vi "Enter Firing Head Info.vi"(7 "error in (no error)":errorcluster) -> (0 "error out":errorcluster, 1 "Abort Test?":bool, 2 "Serial # Out":string, 3 "Model # Out":string)   [LabVIEW 2018]
uses:
  Instrumentation/Door Status Global Variable.vi
panel:
  in  "Model #":string
  in  "Abort Test":bool
  in  "Serial #":string
  in  "Continue":bool
  # "Enter the following information\nfor the firing head:"
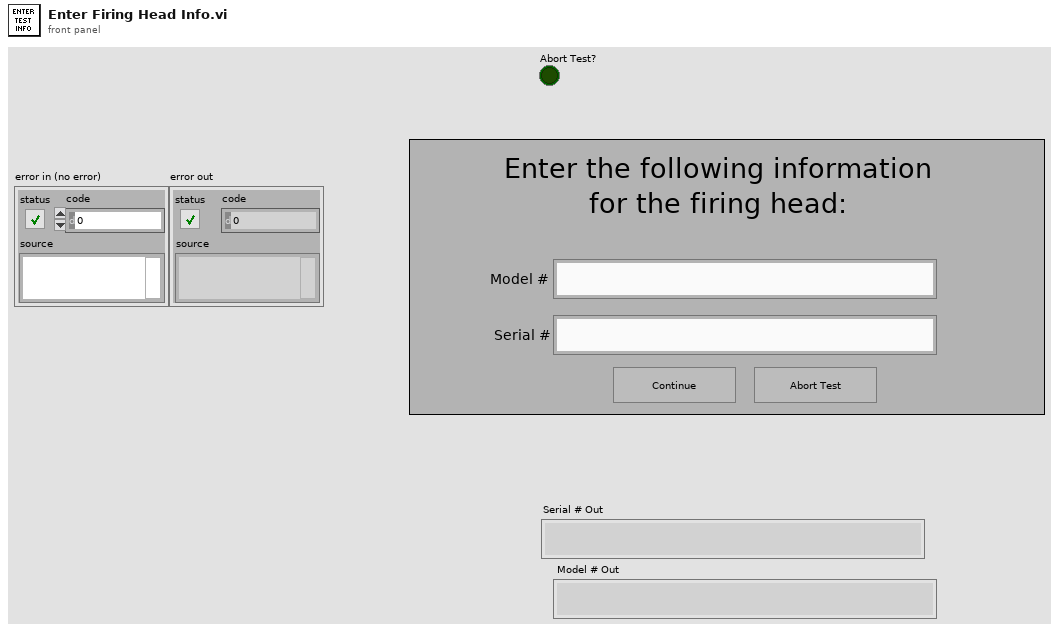
[diagram p1: front panel]
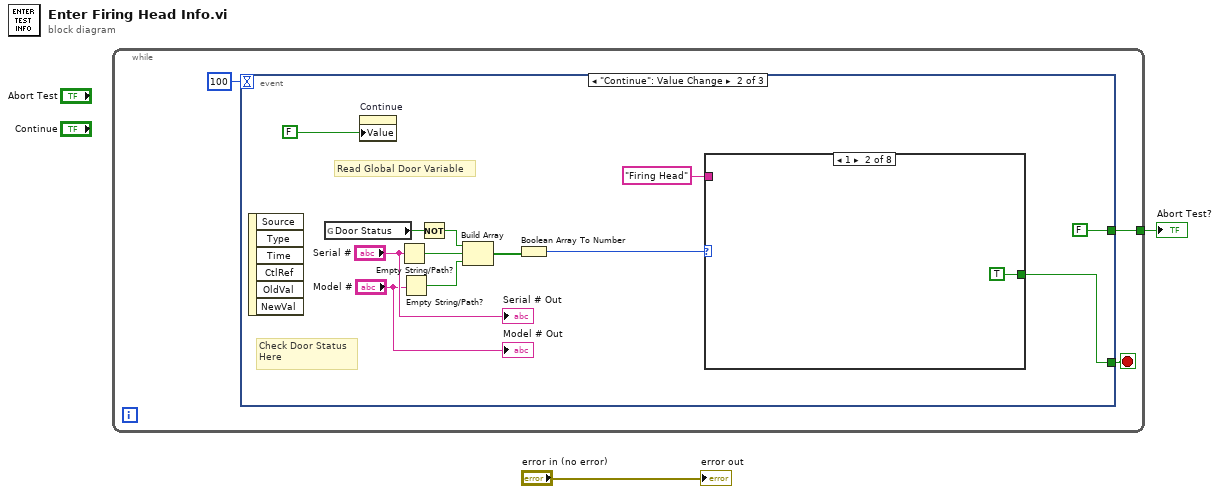
[diagram p0: block diagram]
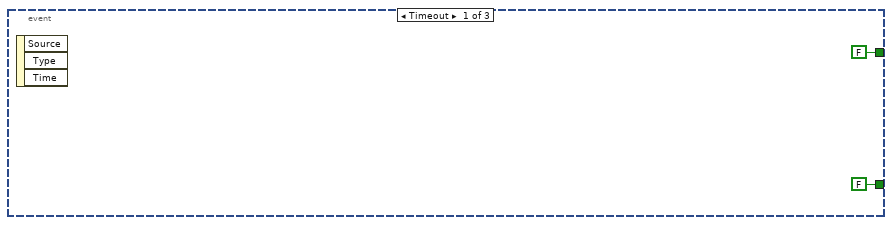
[diagram p2: hidden frame]
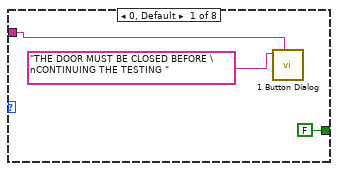
[diagram p3: hidden frame]
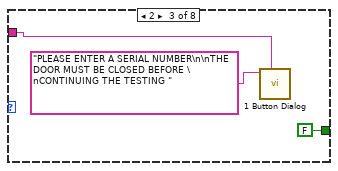
[diagram p4: hidden frame]
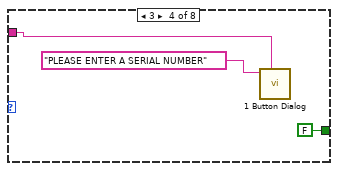
[diagram p5: hidden frame]
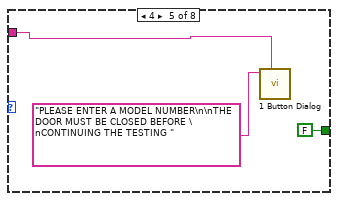
[diagram p6: hidden frame]
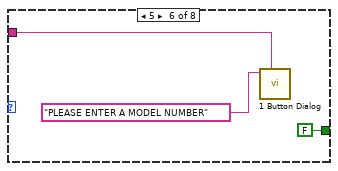
[diagram p7: hidden frame]
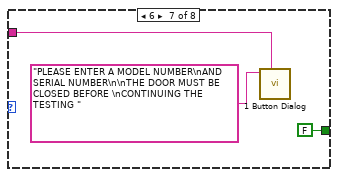
[diagram p8: hidden frame]
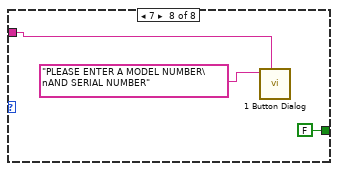
[diagram p9: hidden frame]
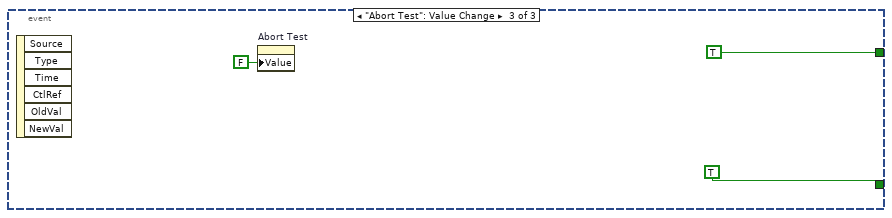
[diagram p10: hidden frame]
diagram:
  n1 = while {
    tunnel: [w4] -> w1
    stop <- w5 stop-if-true
    n2 = event shown="[1] \"Continue\": Value Change" {
      selector: _ -> [_ _ _]
      dyn-events: _ -> [_ _ _]
      timeout: 100 -> [_ _ _]
      tunnel: [FALSE ("Global Stop?") w12 TRUE] -> w5
      tunnel: [FALSE FALSE TRUE] -> w4
      event Timeout {
        n3 = event-data() -> ()  [unwired: 1 in, 3 out]
      }
      event "Continue": Value Change {
        # "Read Global Door Variable"
        # "Check Door Status\nHere"
        n4 = event-data() -> ()  [unwired: 1 in, 6 out]
        n5 = global read "Door Status Global Variable.vi" "Door Status"() -> (w9:bool)
        n6 = property on="Continue" class="Bool (strict)"("Value"=FALSE ("OK")) -> ()  [unwired: 2 in, 2 out]
        n7 = Empty String/Path?(string/path="Serial #") -> (empty?=w14:bool)
        n8 = Empty String/Path?(string/path="Model #") -> (empty?=w13:bool)
        n9 = Not(x=w9) -> (.not. x?=w8:bool)
        n10 = Build Array(w8, w14, w13) -> (w18:bool[])
        n11 = Boolean Array To Number(Boolean array=w18) -> (number=w17:u32)
        n12 = case shown="1" w17 {
          tunnel: [FALSE ("Global Stop?") TRUE ("Global Stop?") FALSE ("Global Stop?") FALSE ("Global Stop?") FALSE ("Global Stop?") FALSE ("Global Stop?") FALSE ("Global Stop?") FALSE ("Global Stop?")] -> w12
          tunnel: "Firing Head" ("Title") -> [w21 _ w25 w28 w31 w34 w37 w40]
          frame 0, Default {
            n13 = call "1 Button Dialog.vi"("Title"=w21, "Dialog Message"="THE DOOR MUST BE CLOSED BEFORE \nCONTINUING THE TESTING ") -> ()  [unwired: 8 in, 2 out]
          }
          frame 1 {
          }
          frame 2 {
            n14 = call "1 Button Dialog.vi"("Title"=w25, "Dialog Message"="PLEASE ENTER A SERIAL NUMBER\n\nTHE DOOR MUST BE CLOSED BEFORE \nCONTINUING THE TESTING ") -> ()  [unwired: 8 in, 2 out]
          }
          frame 3 {
            n15 = call "1 Button Dialog.vi"("Title"=w28, "Dialog Message"="PLEASE ENTER A SERIAL NUMBER") -> ()  [unwired: 8 in, 2 out]
          }
          frame 4 {
            n16 = call "1 Button Dialog.vi"("Title"=w31, "Dialog Message"="PLEASE ENTER A MODEL NUMBER\n\nTHE DOOR MUST BE CLOSED BEFORE \nCONTINUING THE TESTING ") -> ()  [unwired: 8 in, 2 out]
          }
          frame 5 {
            n17 = call "1 Button Dialog.vi"("Title"=w34, "Dialog Message"="PLEASE ENTER A MODEL NUMBER") -> ()  [unwired: 8 in, 2 out]
          }
          frame 6 {
            n18 = call "1 Button Dialog.vi"("Title"=w37, "Dialog Message"="PLEASE ENTER A MODEL NUMBER\nAND SERIAL NUMBER\n\nTHE DOOR MUST BE CLOSED BEFORE \nCONTINUING THE TESTING ") -> ()  [unwired: 8 in, 2 out]
          }
          frame 7 {
            n19 = call "1 Button Dialog.vi"("Title"=w40, "Dialog Message"="PLEASE ENTER A MODEL NUMBER\nAND SERIAL NUMBER") -> ()  [unwired: 8 in, 2 out]
          }
        }
        "Serial # Out" <- "Serial #"
        "Model # Out" <- "Model #"
      }
      event "Abort Test": Value Change {
        n20 = event-data() -> ()  [unwired: 1 in, 6 out]
        n21 = property on="Abort Test" class="Bool (strict)"("Value"=FALSE ("Abort Test")) -> ()  [unwired: 2 in, 2 out]
      }
    }
  }
  "Abort Test?" <- w1
  "error out" <- "error in (no error)"
